vi "Leap Point Position and Velocity.vi"() -> ()   [LabVIEW 2011, in "LVH-Leap.lvlib"]
doc: "This example demonstrates how to read the position and velocity of a point object using the Leap Motion Controller."
uses:
  vi.lib/LabVIEW Hacker/Leap/LVH-Leap.lvlib
  vi.lib/LabVIEW Hacker/Leap/Public/Instance VIs/Read 1 Point Position Velocity.vi
panel:
  out "X Velocity (m/s)":sgl(slide) scale=-2.0..2.0
  out "Y Velocity (m/s)":sgl(slide) scale=2.0..-2.0
  out "Point XZ Position":cluster{"X":sgl, "Y":sgl, "Z":sgl}
  out "Point XZ Position":cluster{"X":sgl, "Z":sgl}[](graph)
  in  "Stop Button":bool
  # "Leap Point Position and Velocity Example\n\nThis example demonstrates how to read the position and velocity of a point object using the Leap Motion Controller.\n\nInstructions\n1. Connect the Leap Motion Controller to the host computer.\n2. Click the Run Arrow.\n3. Position your hand above the Leap Motion controller and extend one finger.  \n4. Notice your finger tip (point) position and velocity indicated on the graph and sliders below."
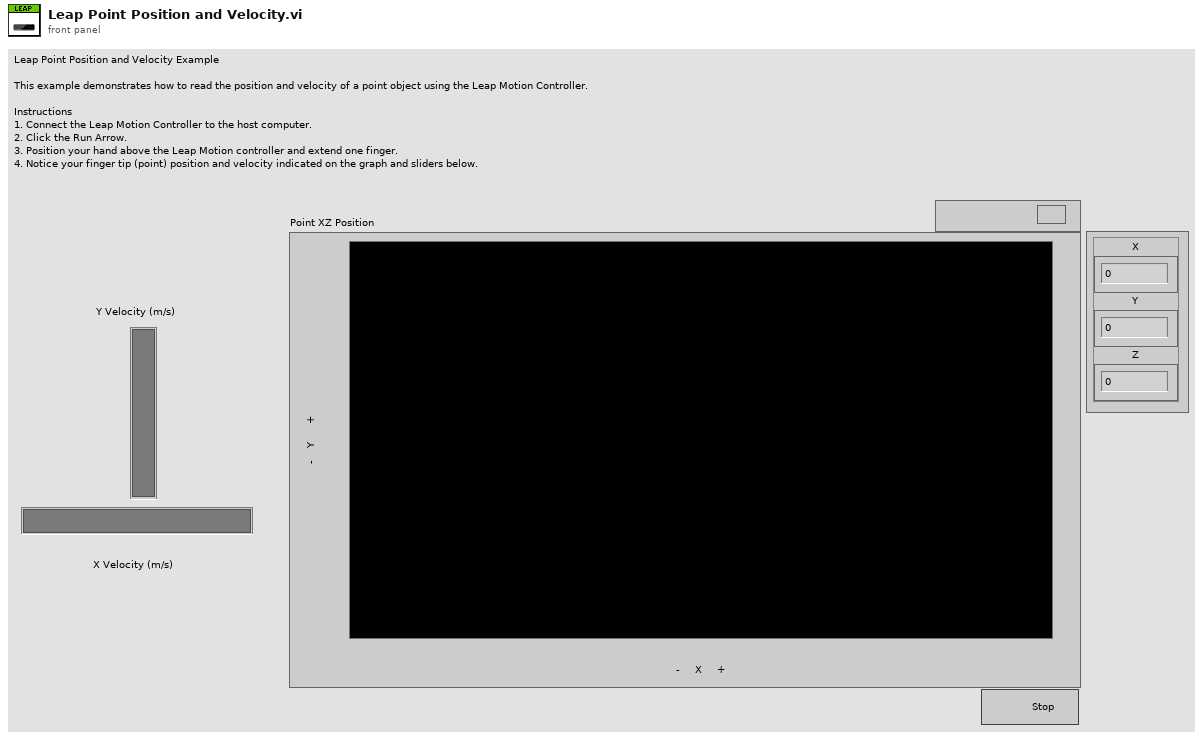
[diagram p1: front panel]
types:
  T1 = typedef "LVH-Leap.lvlib/Leap Handle.ctl" = cluster{"LeapCSharp":refnum<k24>}
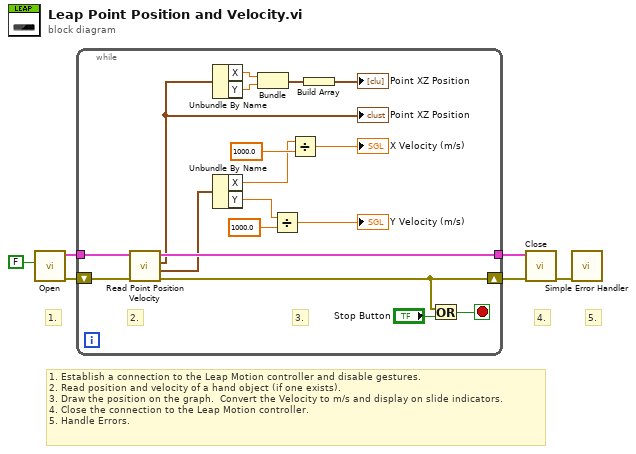
[diagram p0: block diagram]
diagram:
  # "1. Establish a connection to the Leap Motion controller and disable gestures.\n2. Read position and velocity of a hand object (if one exists).\n3. Draw the position on the graph.  Convert the Velocity to m/s and display on slide indicators.\n4. Close the connection to the Leap Motion controller.\n5. Handle Errors."
  # "5."
  # "4."
  # "1."
  n1 = call "Open.vi"("Enable Gestures? (T)"=FALSE) -> ("Error Out"=w4:errorcluster, "Leap Handle"=w6:T1)  [unwired: 9 in]
  n2 = while {
    tunnel: w6 -> [w12]
    shift-right: [w10] -> w5
    shift-left: w4 -> [w9]
    tunnel: [w11] -> w2
    stop <- w24 stop-if-true
    # "3."
    # "2."
    n3 = call-poly "Read Point Position Velocity.vi"("Error In"=w9, "Leap Handle"=w12) -> ("Error Out"=w10:errorcluster, "Point Velocity"=w8:cluster{"X":sgl, "Y":sgl, "Z":sgl}, "Point Position"=w7:cluster{"X":sgl, "Y":sgl, "Z":sgl}, "Leap Handle"=w11:T1)  [unwired: 6 in]
    "Point XZ Position" <- w7
    n4 = Unbundle By Name(w7) -> ("X"=w22:sgl, "Y"=w21:sgl)
    n5 = Unbundle By Name(w8) -> ("X"=w14:sgl, "Y"=w18:sgl)
    n6 = Bundle("X"=w22, "Y"=w21) -> (w20:cluster{"X":sgl, "Y":sgl})  [unwired: 1 in]
    n7 = Divide(x=w18, y=sgl 1000.0) -> (x/y=→"Y Velocity (m/s)":sgl)
    n8 = Divide(x=w14, y=sgl 1000.0) -> (x/y=→"X Velocity (m/s)":sgl)
    n9 = Build Array(w20) -> (→"Point XZ Position":cluster{"X":sgl, "Y":sgl}[])
    n10 = Or(x=w10, y="Stop Button") -> (x .or. y?=w24:bool)
  }
  n11 = call "Close.vi"("Error In"=w5, "Leap Handle"=w2) -> ("Error Out"=w1:errorcluster)  [unwired: 9 in]
  n12 = call <vilib>:"Simple Error Handler.vi"("error in (no error)"=w1) -> ()  [unwired: 4 in, 5 out]
